vi "Enum Dev.vi"(0 "enumfilter":i32, 11 "error in (no error)":errorcluster) -> (2 "DeviceVersion":i32[](array[numeric]), 3 "isBusy":i32[](array[numeric]), 4 "pnDevice":i32, 6 "DevName":string[](array[string]), 8 "SN":string[](array[string]), 10 "UserName":string[](array[string]), 14 "DeviceID":i32[](array[numeric]), 15 "error out":errorcluster)   [LabVIEW 2012, in "AnalogDiscSDKLv.lvlib"]
doc: "extern \"C\" __declspec(dllexport) int Enum_DevLv(ENUMFILTER enumfilter, \n int * pnDevice, char DevName[MAX_DEVICE_NUMBER][DEVICE_INFO_STRING_LENGTH], char SN[MAX_DEVICE_NUMBER][DEVICE_INFO_STRING_LENGTH], char UserName[MAX_DEVICE_NUMBER][DEVICE_INFO_STRING_LENGTH], int isBusy[MAX_DEVICE_NUMBER], DEVID DeviceID[MAX_DEVICE_NUMBER], DEVVER DeviceVersion[MAX_DEVICE_NUMBER] );"
uses:
  <instrlib>/AnalogDiscSDKLv/AnalogDiscSDKLv.lvlib
  <instrlib>/AnalogDiscSDKLv/AnalogDiscSDKLv.dll
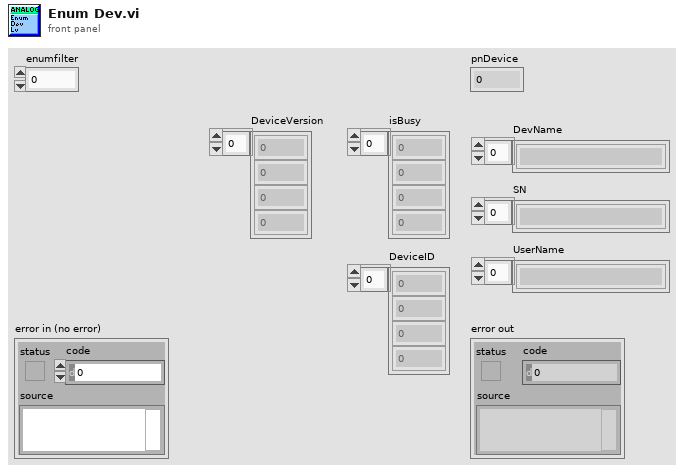
[diagram p1: front panel]
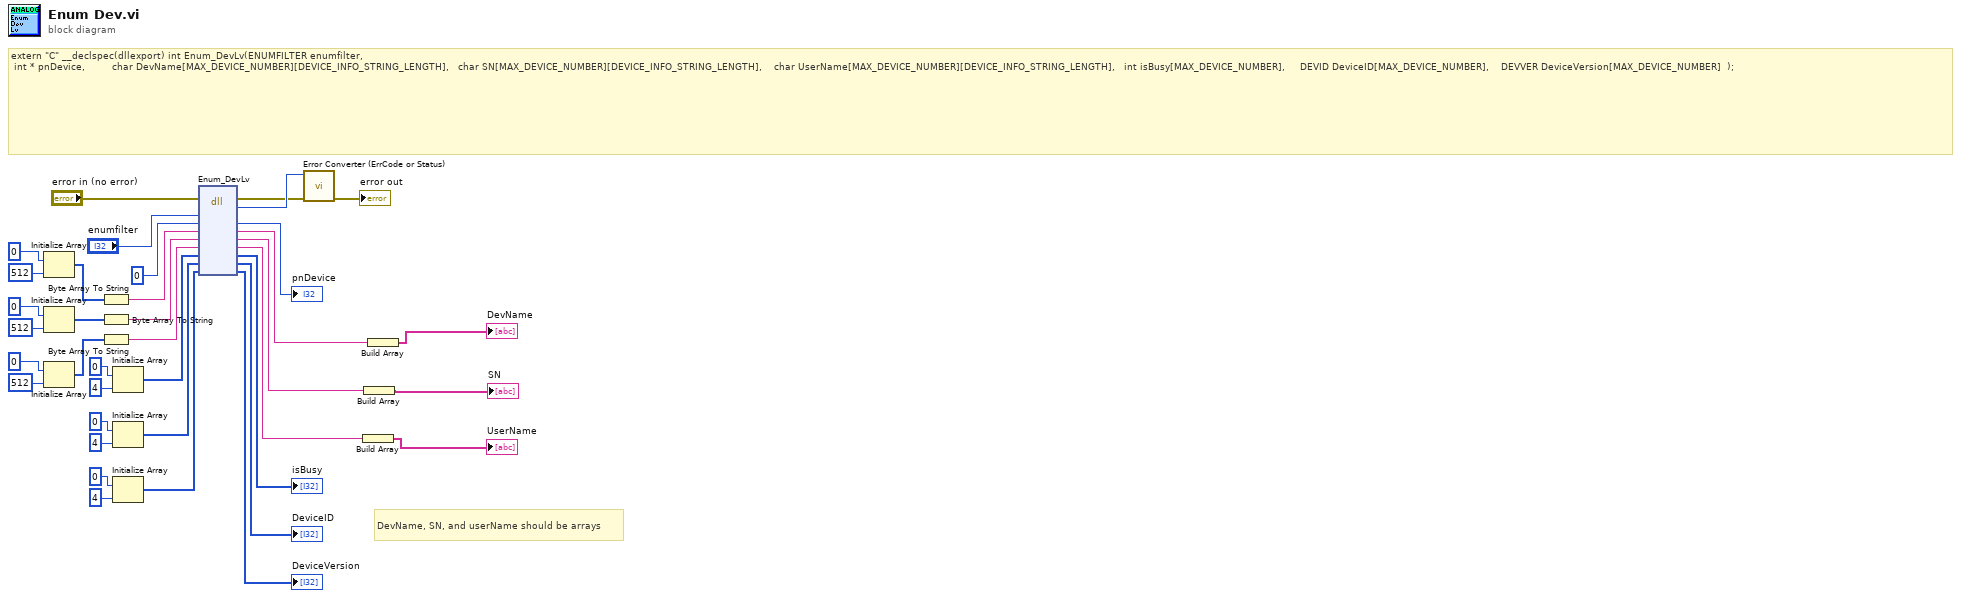
[diagram p0: block diagram]
diagram:
  # "DevName, SN, and userName should be arrays"
  # "extern \"C\" __declspec(dllexport) int Enum_DevLv(ENUMFILTER enumfilter, \n\tint * pnDevice,\t\t\t\t\t\t\t\t\tchar DevName[MAX_DEVICE_NUMBER][DEVICE_INFO_STRING_LENGTH],\t\t\tchar SN[MAX_DEVICE_NUMBER][DEVICE_INFO_STRING_LENGTH],\t\t\t\tchar UserName[MAX_DEVICE_NUMBER][DEVICE_INFO_STRING_LENGTH],\t\t\tint isBusy[MAX_DEVICE_NUMBER],\t\t\t\t\tDEVID DeviceID[MAX_DEVICE_NUMBER],\t\t\t\tDEVVER DeviceVersion[MAX_DEVICE_NUMBER]\t\t);"
  n1 = Initialize Array(u8 0 ("element"), 512 ("dimension size")) -> (w33:u8[])
  n2 = Initialize Array(u8 0 ("element"), 512 ("dimension size")) -> (w28:u8[])
  n3 = Initialize Array(u8 0 ("element"), 512 ("dimension size")) -> (w23:u8[])
  n4 = Byte Array To String(unsigned byte array=w33) -> (string=w32:string)
  n5 = Byte Array To String(unsigned byte array=w28) -> (string=w27:string)
  n6 = Byte Array To String(unsigned byte array=w23) -> (string=w22:string)
  n7 = Initialize Array(0 ("element"), 4 ("dimension size")) -> (w18:i32[])
  n8 = Initialize Array(0 ("element"), 4 ("dimension size")) -> (w14:i32[])
  n9 = Initialize Array(0 ("element"), 4 ("dimension size")) -> (w10:i32[])
  n10 = dll-call lib="C:/Program Files (x86)/National Instruments/LabVIEW 2012/instr.lib/AnalogDiscSDKLv/AnalogDiscSDKLv.*" fn="Enum_DevLv"(error in="error in (no error)", "enumfilter"="enumfilter", "pnDevice"=0, "DevName"=w32, "SN"=w27, "UserName"=w22, "isBusy"=w18, "DeviceID"=w14, "DeviceVersion"=w10) -> (error out=w5:errorcluster, "return type"=w37:i32, "pnDevice"=→"pnDevice":i32, "DevName"=w29:string, "SN"=w24:string, "UserName"=w19:string, "isBusy"=→"isBusy":i32[], "DeviceID"=→"DeviceID":i32[], "DeviceVersion"=→"DeviceVersion":i32[])  [unwired: 3 in, 1 out]
  n11 = call <instrlib>:"Error Converter (ErrCode or Status).vi"("error in (no error)"=w5, "error code"=w37) -> ("error out"=→"error out":errorcluster)  [unwired: 9 in]
  n12 = Build Array(w19) -> (→"UserName":string[])
  n13 = Build Array(w24) -> (→"SN":string[])
  n14 = Build Array(w29) -> (→"DevName":string[])
